vi "ARCO Main Server.vi"() -> ()   [LabVIEW 2017]
uses:
  <vilib>/OPCUA/controls/Data Type.ctl
  <vilib>/OPCUA/controls/Supported Security Policies.ctl
  <vilib>/OPCUA/NI OPC UA Server.lvlib
  <vilib>/OPCUA/NI OPC UA Utility.lvlib
panel:
  out "Result Boolean Control Node":string
  out "Result Numeric Control Node":string
  out "Result Data Node":string
  out "Spoof Boolean Control Node":string
  out "Spoof Numeric Control Node":string
  out "Spoof Data Node":string
  out "Chat Node":string
  out "Boolean Control Action Node":string
  out "Numeric Control Action Node":string
  out "certificate path 2":path
  out "certificate path":path
  out "error out":errorcluster
  out "CIET Data Node":string
  out "server endpoint URL":string
  in  "Stop":bool
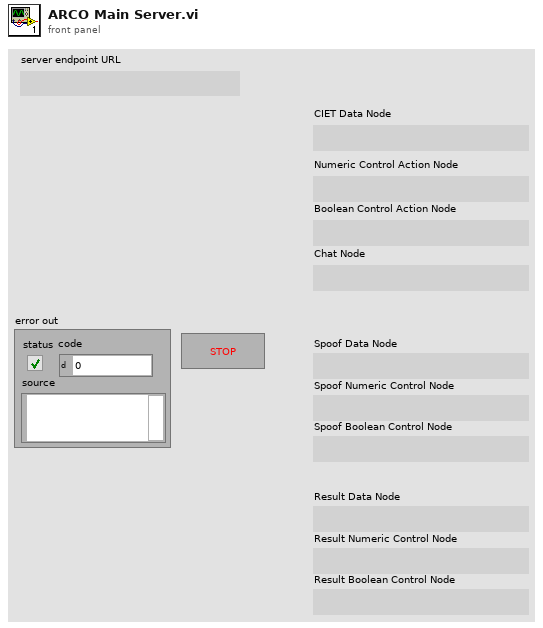
[diagram p1: front panel]
types:
  T1 = typedef "Data Type.ctl" = u16
  T2 = cluster{"name":string, "data type":T1, "access level":u16, "description":string}
  T3 = cluster{"name":string, "data type":T1, "access level 2":u16, "description":string}
  T4 = typedef "Supported Security Policies.ctl" = cluster{"None":bool, "Sign with Basic128Rsa15":bool, "Sign and Encrypt with Basic128Rsa15":bool, "Sign with Basic256":bool, "Sign and Encrypt with Basic256":bool}
  T5 = typedef "OPC UA Server Refnum.ctl" = refnum<k21>
  T6 = typedef "NodeId.ctl" = string
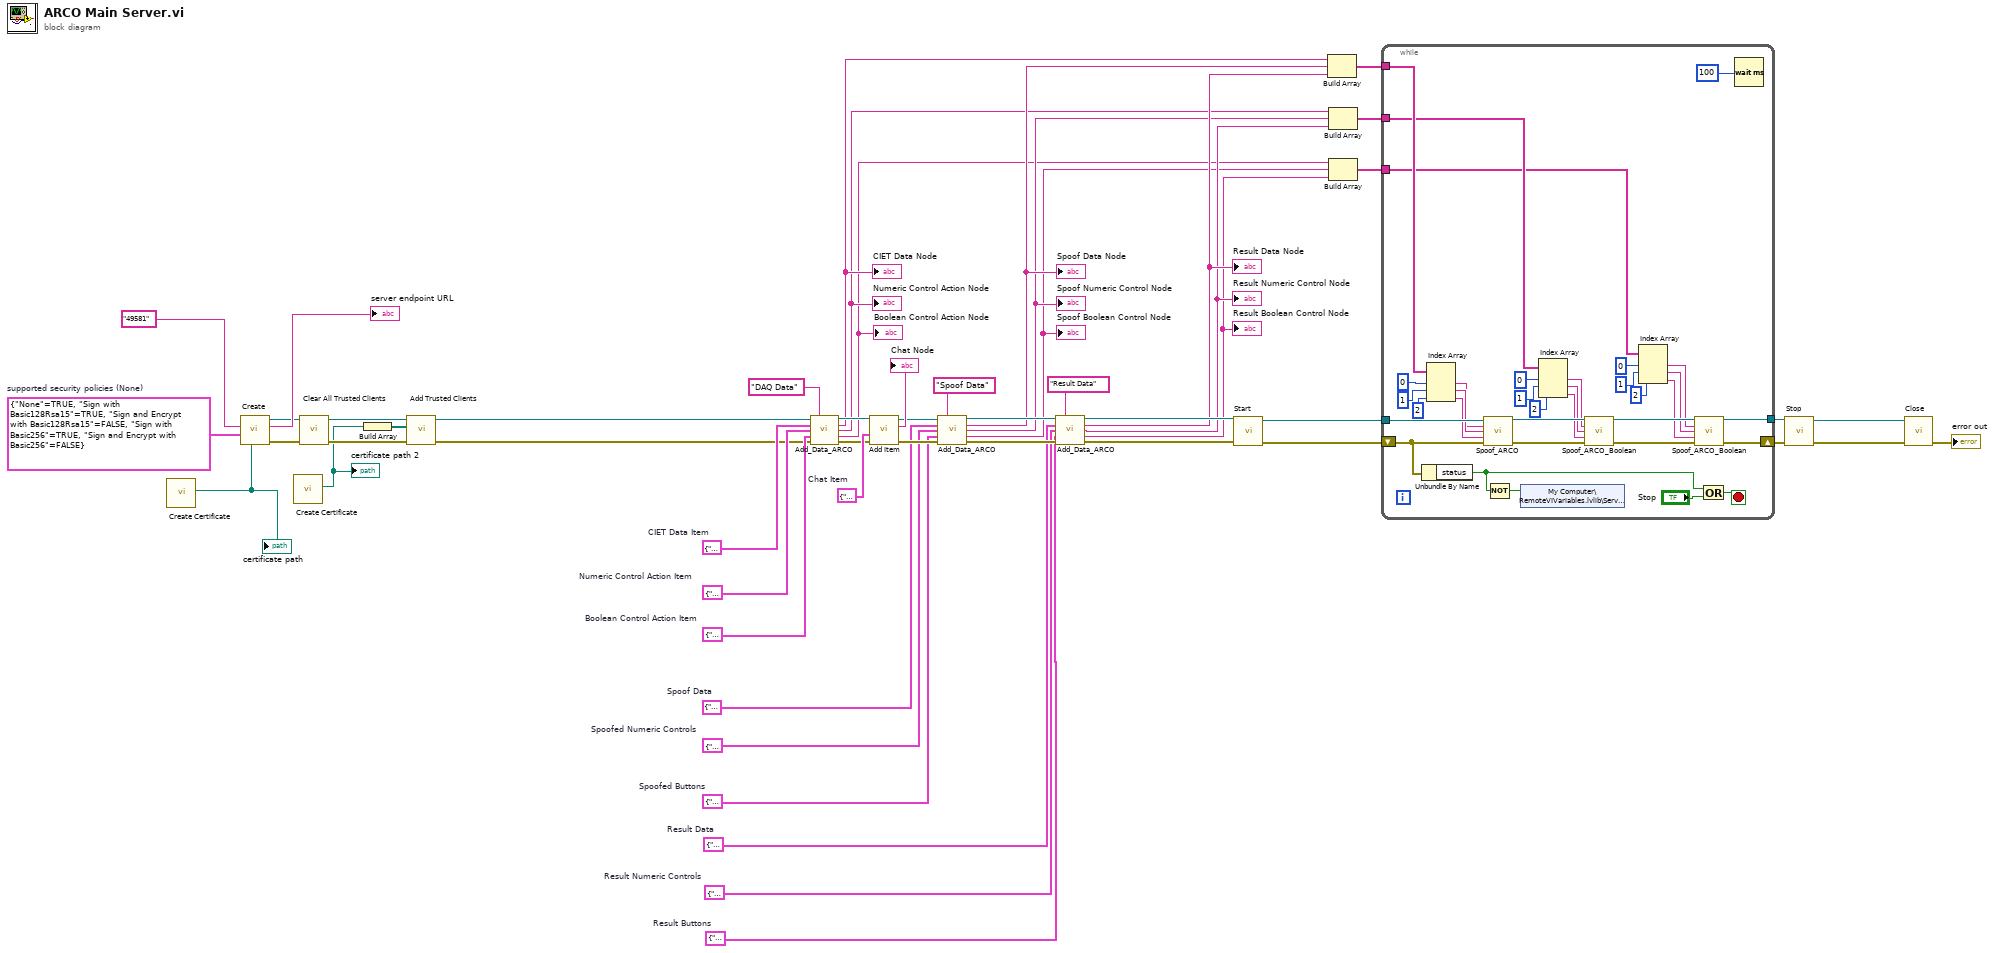
[diagram p0: block diagram]
diagram:
  w17 = T2 {"name"="Spoofed Numeric Controls", "data type"=111, "access level"=3, "description"="Spoofed Setpoints"}  # Spoofed Numeric Controls
  w18 = T2 {"name"="Spoofed CIET Data", "data type"=111, "access level"=3, "description"="Spoofed CIET TC and FM"}  # Spoof Data
  w24 = T2 {"name"="Result Boolean Controls", "data type"=101, "access level"=3, "description"="Result Buttons"}  # Result Buttons
  w25 = T2 {"name"="Result Numeric Controls", "data type"=111, "access level"=3, "description"="Result Setpoints"}  # Result Numeric Controls
  w26 = T3 {"name"="Result CIET Data", "data type"=111, "access level 2"=3, "description"="Result CIET TC and FM"}  # Result Data
  w16 = T2 {"name"="Spoofed Boolean Controls", "data type"=101, "access level"=3, "description"="Spoofed Buttons"}  # Spoofed Buttons
  w38 = T2 {"name"="Chat", "data type"=12, "access level"=3, "description"="Chat"}  # Chat Item
  w34 = T2 {"name"="Boolean Control Actions", "data type"=101, "access level"=3, "description"="Buttons"}  # Boolean Control Action Item
  w35 = T2 {"name"="Numeric Control Actions", "data type"=111, "access level"=3, "description"="Setpoints"}  # Numeric Control Action Item
  w47 = T4 {"None"=TRUE, "Sign with Basic128Rsa15"=TRUE, "Sign and Encrypt with Basic128Rsa15"=FALSE, "Sign with Basic256"=TRUE, "Sign and Encrypt with Basic256"=FALSE}  # supported security policies (None)
  w36 = T2 {"name"="CIET Data", "data type"=111, "access level"=3, "description"="CIET TC and FM"}  # CIET Data Item
  n1 = call <vilib>:"Create Certificate.vi"() -> ("certificate path"=w42:path)  [unwired: 8 in, 3 out]
  "certificate path" <- w42
  n2 = call <vilib>:"Create.vi"("server certificate file"=w42, "supported security policies (None)"=w47, "TCP port (49580)"="49581") -> ("error out"=w43:errorcluster, "server endpoint URL"=→"server endpoint URL":string, "OPC UA server refnum out"=w44:T5)  [unwired: 6 in]
  n3 = call <vilib>:"Create Certificate.vi"() -> ("certificate path"=w41:path)  [unwired: 8 in, 3 out]
  "certificate path 2" <- w41
  n4 = call <vilib>:"Clear All Trusted Clients.vi"("error in (no error)"=w43, "OPC UA server refnum in"=w44) -> ("error out"=w45:errorcluster, "OPC UA server refnum out"=w46:T5)  [unwired: 8 in]
  n5 = Build Array(w41) -> (w40:path[])
  n6 = call <vilib>:"Add Trusted Clients.vi"("error in (no error)"=w45, "trusted client certificates"=w40, "OPC UA server refnum in"=w46) -> ("error out"=w3:errorcluster, "OPC UA server refnum out"=w19:T5)  [unwired: 7 in]
  n7 = call "Add_Data_ARCO.vi"("Refnum in"=w19, "folder name"="DAQ Data", "item 1"=w36, "item 2"=w35, "item 3"=w34, "error in (no error)"=w3) -> ("Refnum out"=w33:T5, "item node ID 1"=w12:string, "item node ID 2"=w9:string, "item node ID 3"=w6:string, "error out"=w32:errorcluster)  [unwired: 5 in]
  "CIET Data Node" <- w12
  "Numeric Control Action Node" <- w9
  "Boolean Control Action Node" <- w6
  n8 = call <vilib>:"Add Item.vi"("error in (no error)"=w32, "item"=w38, "OPC UA server refnum in"=w33) -> ("error out"=w29:errorcluster, "item node ID"=→"Chat Node":T6, "OPC UA server refnum out"=w30:T5)  [unwired: 4 in, 1 out]
  n9 = call "Add_Data_ARCO.vi"("Refnum in"=w30, "folder name"="Spoof Data", "item 1"=w18, "item 2"=w17, "item 3"=w16, "error in (no error)"=w29) -> ("Refnum out"=w27:T5, "item node ID 1"=w11:string, "item node ID 2"=w8:string, "item node ID 3"=w5:string, "error out"=w28:errorcluster)  [unwired: 5 in]
  "Spoof Data Node" <- w11
  "Spoof Numeric Control Node" <- w8
  "Spoof Boolean Control Node" <- w5
  n10 = call "Add_Data_ARCO.vi"("Refnum in"=w27, "folder name"="Result Data", "item 1"=w26, "item 2"=w25, "item 3"=w24, "error in (no error)"=w28) -> ("Refnum out"=w20:T5, "item node ID 1"=w10:string, "item node ID 2"=w7:string, "item node ID 3"=w4:string, "error out"=w21:errorcluster)  [unwired: 5 in]
  "Result Data Node" <- w10
  "Result Numeric Control Node" <- w7
  "Result Boolean Control Node" <- w4
  n11 = call <vilib>:"Start.vi"("error in (no error)"=w21, "OPC UA server refnum in"=w20) -> ("error out"=w2:errorcluster, "OPC UA server refnum out"=w52:T5)  [unwired: 7 in, 1 out]
  n12 = Build Array(w12, w11, w10) -> (w15:string[])
  n13 = Build Array(w9, w8, w7) -> (w14:string[])
  n14 = Build Array(w6, w5, w4) -> (w13:string[])
  n15 = while {
    tunnel: [w84] -> w51
    tunnel: w52 -> [w81]
    tunnel: w15 -> [w62]
    tunnel: w14 -> [w61]
    tunnel: w13 -> [w60]
    shift-right: [w58] -> w1
    shift-left: w2 -> [w57]
    stop <- w56 stop-if-true
    n16 = Unbundle By Name(w57) -> ("status"=w54:bool)
    n17 = Index Array(array=w62, index #1=0, index #2=1, index #3=2) -> (element #1=w75:string, element #2=w76:string, element #3=w77:string)
    n18 = call "Spoof_ARCO.vi"("OPC UA server refnum in"=w81, "DAQ Node"=w75, "Spoof Node"=w76, "Result Node"=w77, "error in (no error)"=w57) -> ("OPC UA server refnum out"=w82:T5, "error out"=w83:errorcluster)  [unwired: 9 in]
    n19 = Not(x=w54) -> (.not. x?=w59:bool)
    n20 = shared-variable "My Computer\\RemoteVIVariables.lvlib\\Server Status"(w59) -> ()  [unwired: 1 in, 1 out]
    n21 = Index Array(array=w61, index #1=0, index #2=1, index #3=2) -> (element #1=w69:string, element #2=w70:string, element #3=w71:string)
    n22 = call "Spoof_ARCO_Boolean.vi"("OPC UA server refnum in"=w82, "Spoof Node"=w69, "DAQ Node"=w70, "Result Node"=w71, "error in (no error)"=w83) -> ("OPC UA server refnum out"=w86:T5, "error out"=w85:errorcluster)  [unwired: 9 in]
    n23 = Index Array(array=w60, index #1=0, index #2=1, index #3=2) -> (element #1=w63:string, element #2=w64:string, element #3=w65:string)
    n24 = call "Spoof_ARCO_Boolean.vi"("OPC UA server refnum in"=w86, "Spoof Node"=w63, "DAQ Node"=w64, "Result Node"=w65, "error in (no error)"=w85) -> ("OPC UA server refnum out"=w84:T5, "error out"=w58:errorcluster)  [unwired: 9 in]
    n25 = Or(x=w54, y="Stop") -> (x .or. y?=w56:bool)
    n26 = Wait (ms)(milliseconds to wait=u32 100) -> ()  [unwired: 1 out]
  }
  n27 = call <vilib>:"Stop.vi"("error in (no error)"=w1, "OPC UA server refnum in"=w51) -> ("error out"=w49:errorcluster, "OPC UA server refnum out"=w50:T5)  [unwired: 8 in]
  n28 = call <vilib>:"Close.vi"("error in (no error)"=w49, "OPC UA server refnum in"=w50) -> ("error out"=→"error out":errorcluster)  [unwired: 9 in]
